vi "main.vi"(8 "error in (no error)":errorcluster, 10 "event":refnum<user-event>, 11 "functional":refnum<user-event>) -> (0 "error out":errorcluster)   [LabVIEW 2015, in "example_01.lvlib" / "light.lvclass"]
uses:
  light.lvclass
  functional/public/_controls/event_functional.ctl
  functional/public/_controls/event_functional_command.ctl
  functional/public/interface/_controls/event_data.ctl
  functional/public/interface/_controls/event_command.ctl
  functional/public/_controls/hmi_references.ctl
  functional/functional.lvlib
  functional/public/interface/interface.lvclass
panel:
  in  "do_it":bool
  out "random_number":dbl
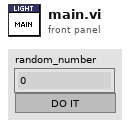
[diagram p1: front panel]
types:
  T1 = typedef "functional.lvlib/hmi_references.ctl" = cluster{"vi_reference":refnum<vi>, "random_number":refnum<vi>, "do_it":refnum<vi>}
  T2 = typedef "functional.lvlib/event_functional_command.ctl" = enum16{"<command_functional>", "--high-level", "stop", "update_hmi_references", "load_interface", "--functional", "do_it", "<null>"}
  T3 = typedef "functional.lvlib/event_functional.ctl" = cluster{"command":T2, "data":variant}
  T4 = typedef "example_01.lvlib/functional.lvlib/interface.lvclass/event_command.ctl" = enum16{"<event_command>", "stop", "<null>"}
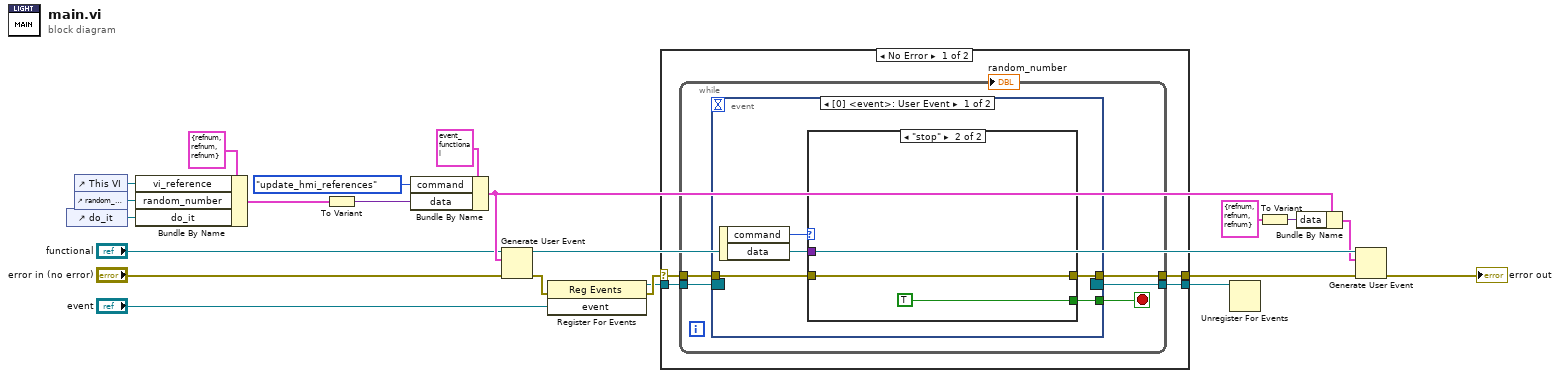
[diagram p0: block diagram]
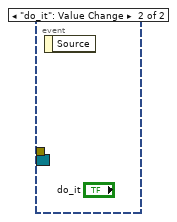
[diagram p3: hidden frame]
diagram:
  n1 = control-ref of="do_it"() -> (w21:refnum<vi>)
  n2 = control-ref of="This VI"() -> (w3:refnum<vi>)
  n3 = control-ref of="random_number"() -> (w2:refnum<vi>)
  n4 = Bundle By Name(cluster=T1 {"vi_reference"=refnum, "random_number"=refnum, "do_it"=refnum} ("hmi_references"), "vi_reference"=w3, "random_number"=w2, "do_it"=w21) -> (w18:T1)
  n5 = To Variant(anything=w18) -> (Variant=w17:variant)
  n6 = Bundle By Name(cluster=T3 {"command"=enum."<command_functional>", "data"=variant} ("event data"), "command"=event_functional_command."update_hmi_references", "data"=w17) -> (w13:T3)
  n7 = Generate User Event(user event="functional", event data cluster=w13, error in="error in (no error)") -> (user event out=w16:refnum<user-event>, error out=w9:errorcluster)  [unwired: 1 in]
  n8 = register-events(error in=w9, "event") -> (reference out=w7:refnum<event-registration>, error out=w8:errorcluster)  [unwired: 1 in]
  n9 = case shown="No Error" w8 {
    selector: w8 -> [w23 w41]
    tunnel: [w26 w41] -> w15
    tunnel: w7 -> [w25 w40]
    tunnel: [w24 w40] -> w6
    frame No Error {
      n10 = while {
        tunnel: w23 -> [w30]
        tunnel: [w29] -> w26
        tunnel: w25 -> [w28]
        tunnel: [w27] -> w24
        stop <- w31 stop-if-true
        n11 = event shown="[0] <event>: User Event" {
          selector: w28 -> [_ _]
          dyn-events: [_ _] -> w27
          timeout: _ -> [_ _]
          tunnel: [w33 _] -> w31
          tunnel: w30 -> [w35 _]
          tunnel: [w32 _] -> w29
          event User Event {
            n12 = event-data() -> ("command"=w36:T4, "data"=w34:variant)  [unwired: 1 in]
            n13 = case shown="\"stop\"" w36 {
              tunnel: w35 -> [w37 w38]
              tunnel: w34 -> [_ _]
              tunnel: [_ TRUE] -> w33
              tunnel: [w37 w38] -> w32
              frame Default {
              }
              frame "stop" {
              }
            }
          }
          event "do_it": Value Change {
            n14 = event-data() -> ()  [unwired: 1 in, 1 out]
          }
        }
      }
    }
    frame Error {
    }
  }
  n15 = Unregister For Events(event registration refnum=w6) -> ()  [unwired: 1 in, 1 out]
  n16 = To Variant(anything=T1 {"vi_reference"=refnum, "random_number"=refnum, "do_it"=refnum} ("hmi_references")) -> (Variant=w11:variant)
  n17 = Bundle By Name(cluster=w13, "data"=w11) -> (w12:T3)
  n18 = Generate User Event(user event=w16, event data cluster=w12, error in=w15) -> (error out=→"error out":errorcluster)  [unwired: 1 in, 1 out]
